vi "LimitAcceleration.vi"(6 "MsPerLoop":u32, 8 "YAxisIn":dbl, 11 "XAxisIn":dbl) -> (0 "YAxisOut":dbl, 3 "XAxisOut":dbl)   [LabVIEW 2013]
panel:
  out "SecToFull":dbl
  out "StepsToFull":dbl
  out "StepsPerSec":dbl
  out "StepSize":dbl
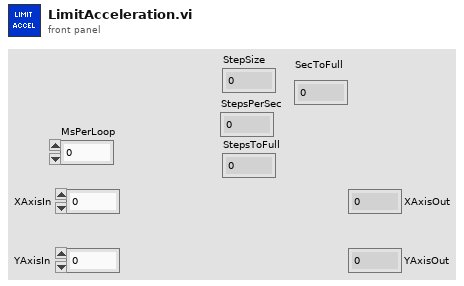
[diagram p1: front panel]
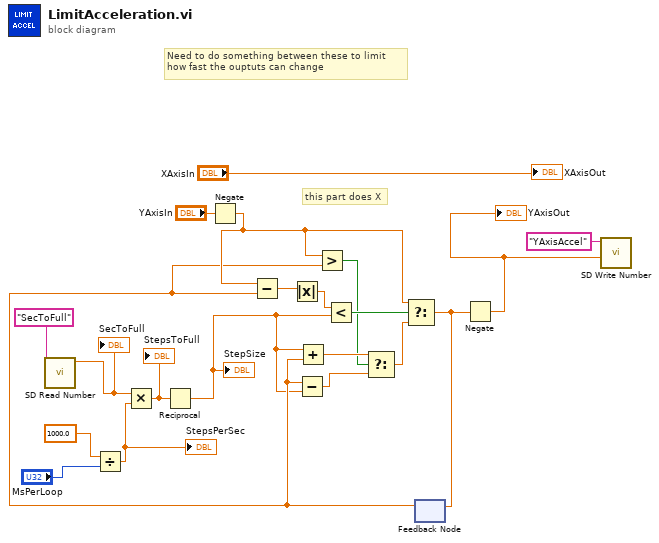
[diagram p0: block diagram]
diagram:
  # "this part does X"
  # "Need to do something between these to limit\nhow fast the ouptuts can change"
  n1 = call <vilib>:"SD Read Number.vi"("Name"="SecToFull") -> ("Numeric"=w1:dbl)  [unwired: 8 in, 2 out]
  "SecToFull" <- w1
  n2 = Divide(x=1000.0, y="MsPerLoop") -> (x/y=w16:dbl)
  "StepsPerSec" <- w16
  n3 = Multiply(x=w1, y=w16) -> (x*y=w15:dbl)
  "StepsToFull" <- w15
  n4 = Reciprocal(x=w15) -> (1/x=w2:dbl)
  "StepSize" <- w2
  n5 = Negate(x="YAxisIn") -> (-x=w8:dbl)
  n6 = feedback #1() -> (w3:dbl)  [unwired: 1 in]
  n7 = Subtract(x=w8, y=w3) -> (x-y=w5:dbl)
  n8 = Absolute Value(x=w5) -> (abs(x)=w4:dbl)
  n9 = Subtract(x=w3, y=w2) -> (x-y=w10:dbl)
  n10 = Add(x=w2, y=w3) -> (x+y=w9:dbl)
  n11 = Greater?(x=w8, y=w3) -> (0:w7:bool)
  n12 = Less?(x=w4, y=w2) -> (x < y?=w20:bool)
  n13 = Select(t=w9, s=w7, f=w10) -> (s? t:f=w6:dbl)
  n14 = Select(t=w8, s=w20, f=w6) -> (s? t:f=w12:dbl)
  n15 = feedback-in #1(w12) -> ()
  n16 = Negate(x=w12) -> (-x=w11:dbl)
  "YAxisOut" <- w11
  n17 = call <vilib>:"SD Write Number.vi"("Numeric"=w11, "Name"="YAxisAccel") -> ()  [unwired: 8 in, 2 out]
  "XAxisOut" <- "XAxisIn"
